vi "measure_current.vi"(8 "error in":errorcluster, 10 "Measurement settings":T1={"Start Wavelength (nm)"=300.0, "End Wavelength (nm)"=900.0, "Increment (nm)"=5.0, "White Bias (No. of Suns)"=1.0, "Averages per wavlength"=1.0, "Sensitivity"=17} {"Sensitivity" items=["Auto Gain"=-1, "2 nV/fA"=0, "5 nV/fA"=1, "10 nV/fA"=2, "20 nV/fA"=3, "50 nV/fA"=4, "100 nV/fA"=5, "200 nV/fA"=6, "500 nV/fA"=7, "1 uV/pA"=8, "2 uV/pA"=9, "5 uV/pA"=10, "10 uV/pA"=11, "20 uV/pA"=12, "50 uV/pA"=13, "100 uV/pA"=14, "200 uV/pA"=15, "500 uV/pA"=16, "1 mV/nA"=17, "2 mV/nA"=18, "5 mV/nA"=19, "10 mV/nA"=20, "20 mV/nA"=21, "50 mV/nA"=22, "100 mV/nA"=23, "200 mV/nA"=24, "500 mV/mA"=25, "1 V/uA"=26]; "Averages per wavlength" format="%#.2f"; "White Bias (No. of Suns)" format="%#.2f"; "End Wavelength (nm)" format="%#.2f"; "Start Wavelength (nm)" format="%#.2f"}, 11 "VISA resource name in":refnum<visa-resource-name>="GPIB0::8::INSTR") -> (0 "error out":errorcluster, 3 "Measurement in mA":dbl)   [LabVIEW 2016]
uses:
  typedefs/measurement_settings.ctl
  <instrlib>/Stanford Research 830/Public/Data/Read (1 Parameter).vi
  <instrlib>/Stanford Research 830/Stanford Research 830.lvlib
panel:
  out "Measurement in V":dbl
  out "Averaged current (mA)":dbl
  out "Intensity-graph":T2(graph)
  in  "Parameter (1: X)":u16(ring)=3 items=["X"=1, "Y"=2, "R"=3, "Theta"=4, "Channel 1"=5, "Channel 2"=6, "Aux In 1"=7, "Aux In 2"=8, "Aux In 3"=9, "Aux In 4"=10]
  out "VISA resource name out":refnum<visa-resource-name>
  # "Wavelength average intensity"
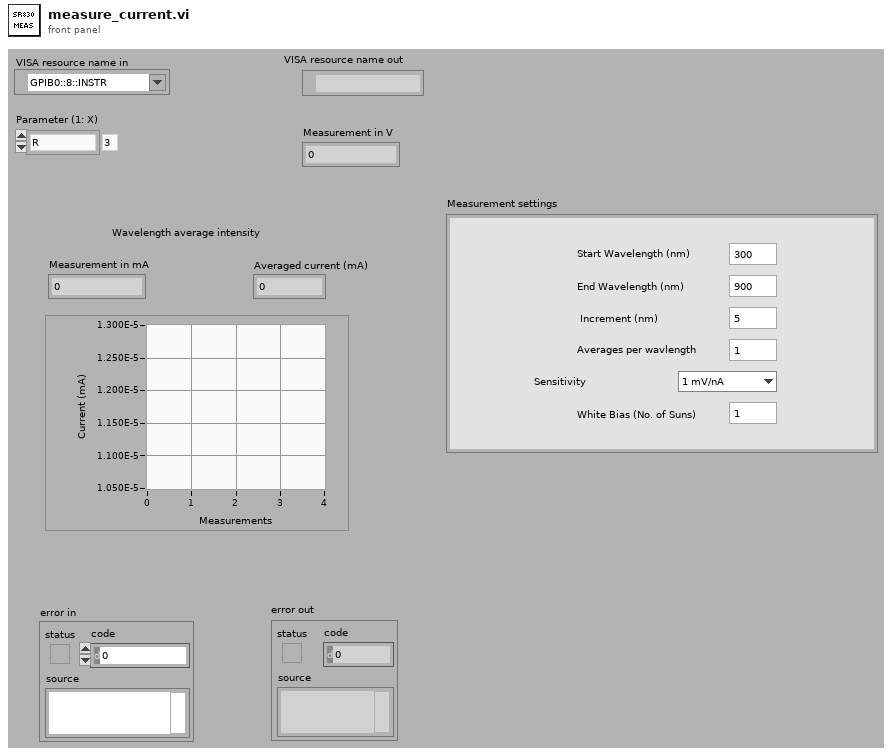
[diagram p1: front panel]
types:
  T1 = typedef "measurement_settings.ctl" = cluster{"Start Wavelength (nm)":dbl, "End Wavelength (nm)":dbl, "Increment (nm)":dbl, "White Bias (No. of Suns)":dbl, "Averages per wavlength":dbl, "Sensitivity":i16}
  T2 = cluster{"meas_index 2":i32[], "Intensity 3":dbl[]}
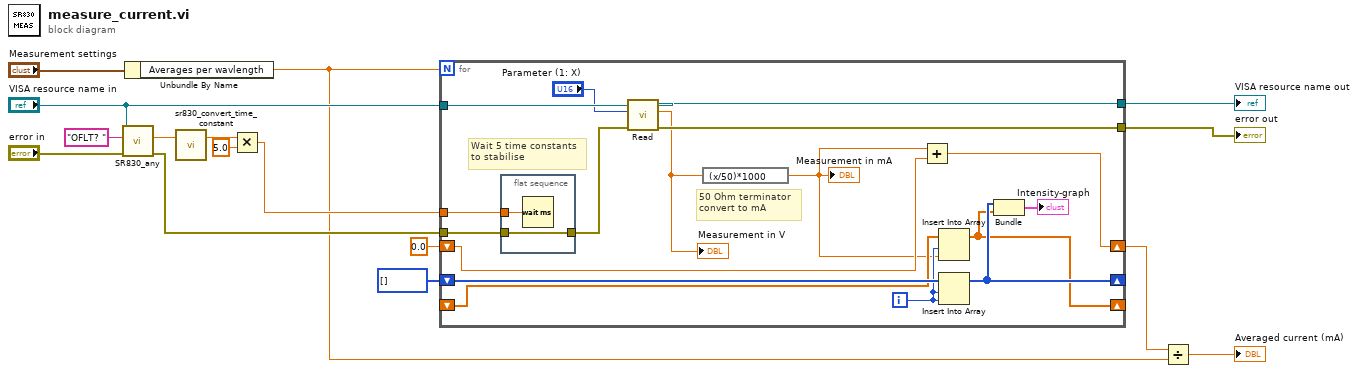
[diagram p0: block diagram]
diagram:
  n1 = call "SR830_any.vi"("error in (no error)"="error in", "initial string"="OFLT? ", "VISA resource name"="VISA resource name in") -> ("error out"=w6:errorcluster, "Measurement"=w7:dbl)  [unwired: 6 in, 1 out]
  n2 = Unbundle By Name("Measurement settings") -> ("Averages per wavlength"=w1:dbl)
  n3 = call "sr830_convert_time_constant.vi"("Time constant code"=w7) -> ("time constant  in ms"=w13:dbl)  [unwired: 2 in]
  n4 = Multiply(x=w13, y=5.0) -> (x*y=w11:dbl)
  n5 = for {
    N: w1 -> [_]
    tunnel: "VISA resource name in" -> [w33]
    tunnel: [w32] -> w15
    tunnel: [w31] -> w14
    shift-right: [w25] -> w5
    shift-left: 0.0 -> [w22]
    shift-right: [w24] -> _
    shift-left: i32[] [] -> [w29]
    shift-right: [w23] -> _
    shift-left: _ -> [w28]
    tunnel: w11 -> [w21]
    tunnel: w6 -> [w20]
    i -> [w27]
    # "50 Ohm terminator\nconvert to mA"
    # "Wait 5 time constants\nto stabilise"
    n6 = flat-sequence {
      tunnel: w21 -> [w35]
      tunnel: w20 -> [w34]
      tunnel: [w34] -> w19
      frame #0 {
        n7 = Wait (ms)(milliseconds to wait=w35) -> ()  [unwired: 1 out]
      }
    }
    n8 = call-poly <instrlib>:"Read.vi"("error in (no error)"=w19, "Parameter (1: X)"="Parameter (1: X)", "VISA resource name"=w33) -> ("error out"=w31:errorcluster, "Measurement"=w17:dbl, "VISA resource name out"=w32:refnum<visa-resource-name>)  [unwired: 6 in]
    "Measurement in V" <- w17
    n9 = expression code="(x/50)*1000"(w17) -> (w18:dbl)
    "Measurement in mA" <- w18
    n10 = Add(x=w18, y=w22) -> (x+y=w25:dbl)
    n11 = Insert Into Array(array=w28, index=w27, new element=w18) -> (w23:dbl[])
    n12 = Insert Into Array(array=w29, index=w27, new element=w27) -> (w24:i32[])
    n13 = Bundle(w24, w23) -> (→"Intensity-graph":cluster{i32[], dbl[]})  [unwired: 1 in]
  }
  "VISA resource name out" <- w15
  "error out" <- w14
  n14 = Divide(x=w5, y=w1) -> (x/y=→"Averaged current (mA)":dbl)
